vi "P4CMD Provider Supports Functionality.vi"(8 "error in (no error)":errorcluster, 10 "functionality":T1) -> (0 "error out":errorcluster, 2 "provider supports?":bool)   [LabVIEW 2017, in "NI_SCC_P4CMD.lvlib"]
uses:
  <vilib>/SourceControl/Providers/P4CMD/NI_SCC_P4CMD.lvlib
  <vilib>/SourceControl/sccapi/SCCAPI SCC Provider Functionality.ctl
  <vilib>/SourceControl/sccapi/NI_SCC.lvlib
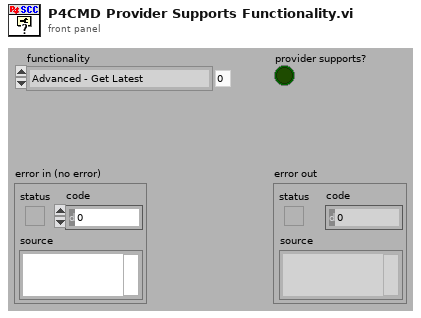
[diagram p1: front panel]
types:
  T1 = typedef "NI_SCC.lvlib/SCCAPI SCC Provider Functionality.ctl" = enum16{"Advanced - Get Latest", "Advanced - CheckOut", "Advanced - CheckIn", "Advanced - UndoCheckOut", "Advanced - Add", "Advanced - Remove", "Advanced - FileCompare", "Advanced - FileHistory", "Advanced - FileProperties", "Advanced - ConfigOptions", "Run SCC", "Configure Project", "Comment on CheckOut", "Comment on CheckIn", "Comment on Add", "Comment on Remove", "Keep Checked Out", "Get File Copy", "Multifile History"}
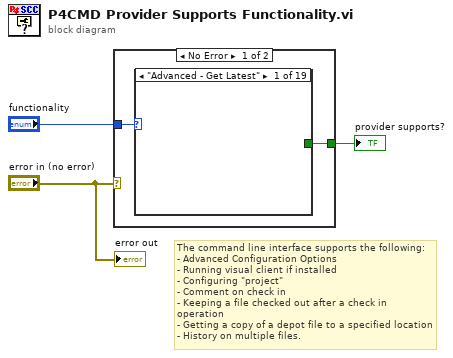
[diagram p0: block diagram]
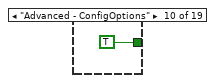
[diagram p10: hidden frame]
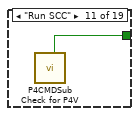
[diagram p11: hidden frame]
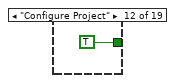
[diagram p12: hidden frame]
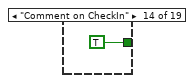
[diagram p14: hidden frame]
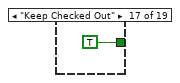
[diagram p17: hidden frame]
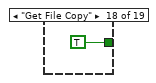
[diagram p18: hidden frame]
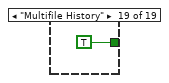
[diagram p19: hidden frame]
diagram:
  # "The command line interface supports the following:\n- Advanced Configuration Options\n- Running visual client if installed\n- Configuring \"project\"\n- Comment on check in\n- Keeping a file checked out after a check in operation\n- Getting a copy of a depot file to a specified location\n- History on multiple files."
  n1 = case shown="No Error" "error in (no error)" {
    tunnel: [w4 _] -> w3
    tunnel: "functionality" -> [w5 _]
    frame No Error {
      n2 = case shown="\"Advanced - Get Latest\"" w5 {
        tunnel: [_ _ _ _ _ _ _ _ _ TRUE ("provider supports?") w7 TRUE ("provider supports?") _ TRUE ("provider supports?") _ _ TRUE ("provider supports?") TRUE ("provider supports?") TRUE ("provider supports?")] -> w4
        frame "Advanced - Get Latest" {
        }
        frame "Advanced - CheckOut" {
        }
        frame "Advanced - CheckIn" {
        }
        frame "Advanced - UndoCheckOut" {
        }
        frame "Advanced - Add" {
        }
        frame "Advanced - Remove" {
        }
        frame "Advanced - FileCompare" {
        }
        frame "Advanced - FileHistory" {
        }
        frame "Advanced - FileProperties" {
        }
        frame "Advanced - ConfigOptions" {
        }
        frame "Run SCC" {
          n3 = call <vilib>:"P4CMDSub Check for P4V.vi"() -> ("visual client found?"=w7:bool)  [unwired: 9 in, 2 out]
        }
        frame "Configure Project" {
        }
        frame "Comment on CheckOut" {
        }
        frame "Comment on CheckIn" {
        }
        frame "Comment on Add" {
        }
        frame "Comment on Remove" {
        }
        frame "Keep Checked Out" {
        }
        frame "Get File Copy" {
        }
        frame "Multifile History" {
        }
      }
    }
    frame Error {
    }
  }
  "provider supports?" <- w3
  "error out" <- "error in (no error)"
